vi "create.vi"(8 "error in":errorcluster) -> (0 "error out":errorcluster, 3 "stream publisher out":refnum<class "publisher.lvclass">)   [LabVIEW 2013, in "data stream.lvlib" / "publisher.lvclass"]
uses:
  publisher.lvclass
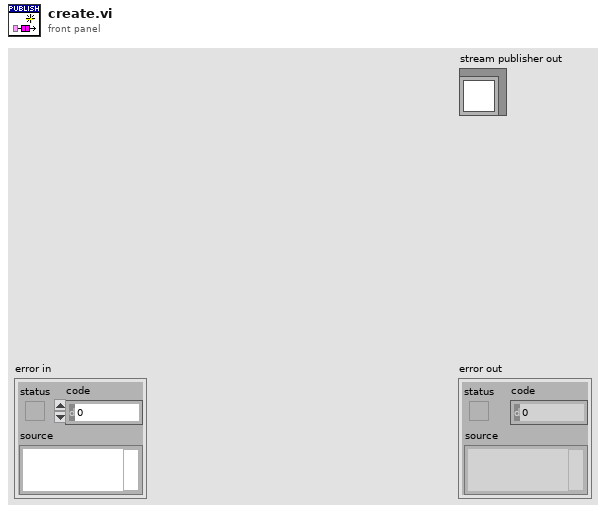
[diagram p1: front panel]
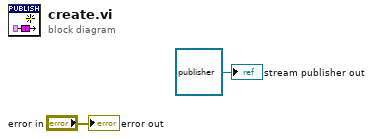
[diagram p0: block diagram]
diagram:
  "error out" <- "error in"
  "stream publisher out" <- refnum<class "publisher.lvclass"> refnum ("stream publisher out")
